vi "PicoScope3000aGetRapidBlock.vi"(0 "error in":errorcluster, 5 "Number of Segments":u32, 7 "handle in":i16, 9 "Device Info":T1, 11 "Rapid Block Acquisition Settings":T2 {"Down Sample Ratio" min=1 step=1; "Down-Sample Mode" items=["None", "Aggregate", "Decimate", "Average"]}) -> (2 "Channel A Buffer":i16[][](array[numeric]), 3 "Channel B Buffer":i16[][](array[numeric]), 4 "error out":errorcluster, 6 "handle out":i16, 8 "noOfSamples Array":u32[](array[numeric]), 10 "Port 0 Buffer":i16[][](array[numeric]), 12 "Overflow":i16[](array[numeric]), 13 "Channel C Buffer":i16[][](array[numeric]), 14 "Channel D Buffer":i16[][](array[numeric]), 15 "Port 1 Buffer":i16[][](array[numeric]))   [LabVIEW 2009]
doc: "This VI gets a set of blocks captured using rapid block mode. It outputs two-dimensional arrays for each channel that contain data from all the requested captures."
uses:
  ps3000a.dll
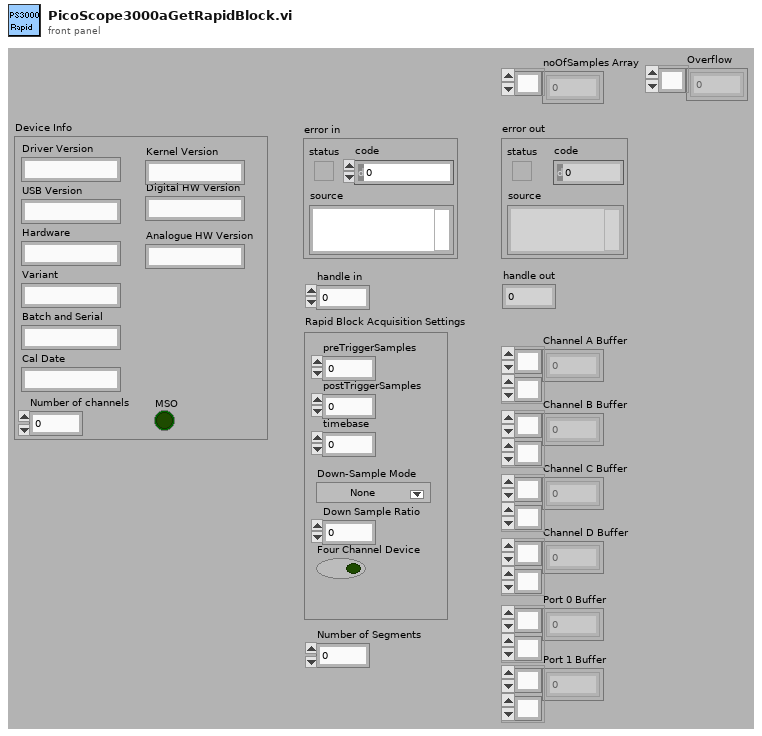
[diagram p1: front panel]
types:
  T1 = cluster{"Driver Version":string, "USB Version":string, "Hardware":string, "Variant":string, "Batch and Serial":string, "Cal Date":string, "Kernel Version":string, "Digital HW Version":string, "Analogue HW Version":string, "MSO":bool, "Number of channels":i16}
  T2 = cluster{"preTriggerSamples":u32, "postTriggerSamples":u32, "timebase":u32, "Down-Sample Mode":i32, "Down Sample Ratio":u32, "Four Channel Device":bool}
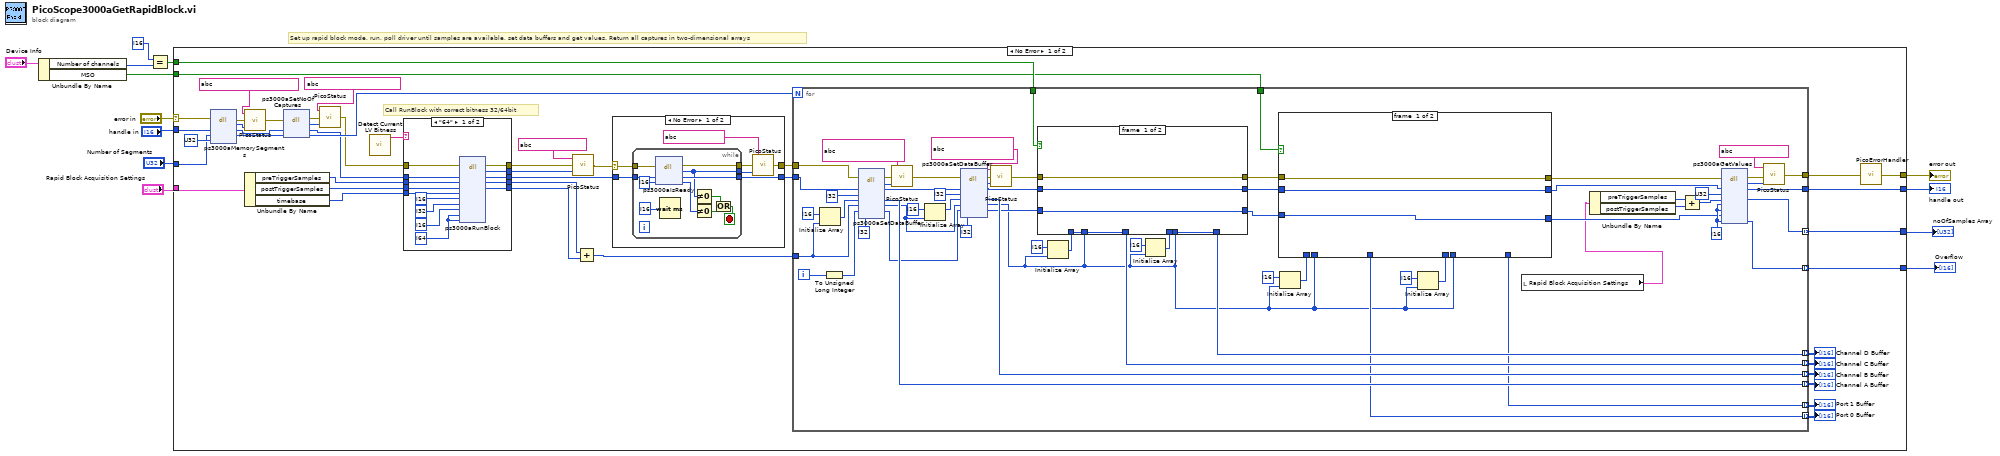
[diagram p0: block diagram]
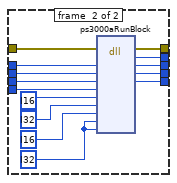
[diagram p2: hidden frame]
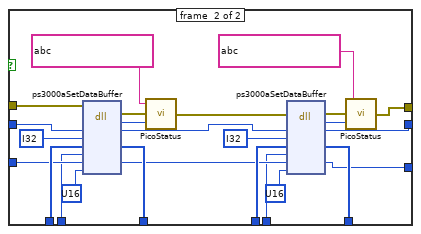
[diagram p3: hidden frame]
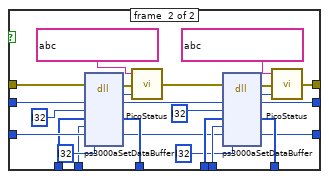
[diagram p4: hidden frame]
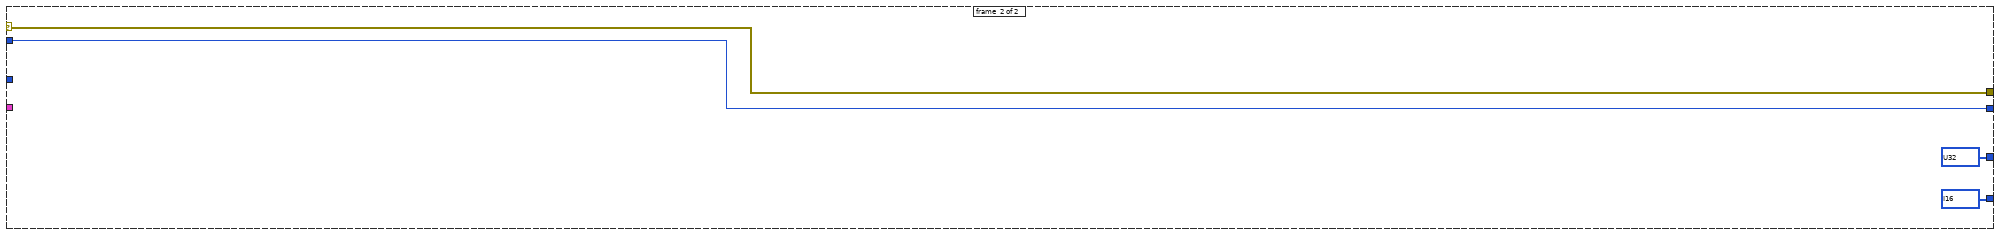
[diagram p6: hidden frame]
diagram:
  # "Set up rapid block mode, run, poll driver until samples are available, set data buffers and get values. Return all captures in two-dimensional arrays"
  n1 = Unbundle By Name("Device Info") -> ("Number of channels"=w8:i16, "MSO"=w5:bool)
  n2 = Equal?(x=i16 ?, y=w8) -> (x = y?=w6:bool)
  n3 = case shown="No Error" "error in" {
    selector: "error in" -> [w53 w229]
    tunnel: [w33 w229] -> w12
    tunnel: "handle in" -> [w52 w228]
    tunnel: [w35 w228] -> w10
    tunnel: [w30 u32[] ?] -> w2
    tunnel: w6 -> [w29 _]
    tunnel: w5 -> [w28 _]
    tunnel: "Rapid Block Acquisition Settings" -> [w27 _]
    tunnel: "Number of Segments" -> [w26 _]
    tunnel: [w14 i16[] ?] -> w1
    frame #0 {
      # "Call RunBlock with correct bitness 32/64bit"
      n4 = dll-call lib="ps3000a.dll" fn="ps3000aMemorySegments" ("ps3000.dll:_ps3000_open_unit@0")(error in=w53, "handle"=w52, "nSegments"=w26, "nMaxSamples"=u32 ?) -> (error out=w50:errorcluster, "PICO_STATUS"=w51:i32, "handle"=w46:i16, "nSegments"=w47:u32)  [unwired: 3 in, 1 out]
      n5 = Unbundle By Name(w27) -> ("preTriggerSamples"=w17:u32, "postTriggerSamples"=w16:u32, "timebase"=w15:u32)
      n6 = call "PicoStatus.vi"("PICO STATUS"=w51, "error in"=w50, "source"=string ?) -> ("error out"=w45:errorcluster)
      n7 = dll-call lib="ps3000a.dll" fn="ps3000aSetNoOfCaptures" ("ps3000.dll:_ps3000_open_unit@0")(error in=w45, "handle"=w46, "nCaptures"=w47) -> (error out=w43:errorcluster, "PICO_STATUS"=w44:i32, "handle"=w18:i16, "nCaptures"=w40:u32)  [unwired: 2 in, 1 out]
      n8 = call "PicoStatus.vi"("PICO STATUS"=w44, "error in"=w43, "source"=string ?) -> ("error out"=w20:errorcluster)
      n9 = call "Detect Current LV Bitness.vi"() -> ("bitness"=w19:string)  [unwired: 11 in]
      n10 = case shown="\"64\"" w19 {
        tunnel: [w71 w85] -> w23
        tunnel: [w70 w84] -> w22
        tunnel: [w69 w83] -> w21
        tunnel: w15 -> [w68 w82]
        tunnel: w17 -> [w67 w81]
        tunnel: w16 -> [w66 w80]
        tunnel: [w65 w79] -> w24
        tunnel: [w64 w78] -> w25
        tunnel: w20 -> [w63 w77]
        tunnel: w18 -> [w62 w76]
        frame #0 {
          w58 = i64 ? ("pParameter")
          n11 = dll-call lib="ps3000a.dll" fn="ps3000aRunBlock" ("ps3000.dll:_ps3000_open_unit@0")(error in=w63, "handle"=w62, "preTriggerSamples"=w67, "postTriggerSamples"=w66, "timebase"=w68, "oversample"=i16 ?, "timeindisposed"=i32 ? ("pParameter"), "segmentIndex"=i16 ? ("pParameter"), "lpReady"=w58, "pParameter"=w58) -> (error out=w64:errorcluster, "PICO_STATUS"=w65:i32, "handle"=w71:i16, "preTriggerSamples"=w70:u32, "postTriggerSamples"=w69:u32)  [unwired: 8 in, 1 out]
        }
        frame #1 {
          w72 = i32 ? ("pParameter")
          n12 = dll-call lib="ps3000a.dll" fn="ps3000aRunBlock" ("ps3000.dll:_ps3000_open_unit@0")(error in=w77, "handle"=w76, "preTriggerSamples"=w81, "postTriggerSamples"=w80, "timebase"=w82, "oversample"=i16 ?, "timeindisposed"=i32 ? ("pParameter"), "segmentIndex"=i16 ? ("pParameter"), "lpReady"=w72, "pParameter"=w72) -> (error out=w78:errorcluster, "PICO_STATUS"=w79:i32, "handle"=w85:i16, "preTriggerSamples"=w84:u32, "postTriggerSamples"=w83:u32)  [unwired: 8 in, 1 out]
        }
      }
      n13 = call "PicoStatus.vi"("PICO STATUS"=w24, "error in"=w25, "source"=string ?) -> ("error out"=w55:errorcluster)
      n14 = Add(x=w22, y=w21) -> (x+y=w41:u32)
      n15 = case shown="No Error" w55 {
        selector: w55 -> [w210 w224]
        tunnel: w23 -> [w212 w225]
        tunnel: [w211 w225] -> w57
        tunnel: [w209 w224] -> w56
        frame #0 {
          n16 = while {
            tunnel: [w223] -> w211
            tunnel: w212 -> [w222]
            tunnel: [w217] -> w207
            tunnel: w210 -> [w216]
            tunnel: [w215] -> w208
            stop <- w221 stop-if-true
            n17 = dll-call lib="ps3000a.dll" fn="ps3000aIsReady" ("ps3000.dll:_ps3000_open_unit@0")(error in=w216, "handle"=w222, "ready"=i16 ?) -> (error out=w215:errorcluster, "status"=w217:i32, "handle"=w223:i16, "ready"=w218:i16)  [unwired: 2 in, 1 out]
            n18 = Wait (ms)(milliseconds to wait=i16 ? ("ready")) -> ()  [unwired: 1 out]
            n19 = Not Equal To 0?(x=w217) -> (x != 0?=w219:bool)
            n20 = Not Equal To 0?(x=w218) -> (x != 0?=w220:bool)
            n21 = Or(x=w219, y=w220) -> (x .or. y?=w221:bool)
          }
          n22 = call "PicoStatus.vi"("PICO STATUS"=w207, "error in"=w208, "source"=string ?) -> ("error out"=w209:errorcluster)
        }
        frame #1 {
        }
      }
      n23 = for {
        N: w40 -> [_]
        tunnel: w57 -> [w147]
        tunnel: w56 -> [w140]
        tunnel: w29 -> [w129]
        tunnel: [w132] -> w39 mode=indexing
        tunnel: [w131] -> w38 mode=indexing
        tunnel: [w110] -> w37 mode=indexing
        tunnel: [w128] -> w36 mode=indexing
        tunnel: w41 -> [w130]
        tunnel: [w119] -> w35
        tunnel: [w105] -> w34
        tunnel: w28 -> [w104]
        tunnel: [w95] -> w32 mode=indexing
        tunnel: [w94] -> w31 mode=indexing
        tunnel: [w88] -> w30 mode=indexing
        tunnel: [w86] -> w14 mode=indexing
        i -> [w90]
        w127 = i16 ? ("overflow")
        n24 = Initialize Array(i16 ? ("element"), w130) -> (w146:i16[])
        n25 = To Unsigned Long Integer(number=w90) -> (unsigned 32bit integer=w89:u32)
        n26 = dll-call lib="ps3000a.dll" fn="ps3000aSetDataBuffer" ("ps3000.dll:_ps3000_open_unit@0")(error in=w140, "handle"=w147, "channel"=i32 ?, "buffer"=w146, "bufferLth"=w130, "waveform"=w89, "downSampleRatioMode"=i32 ?) -> (error out=w138:errorcluster, "PICO_STATUS"=w139:i32, "handle"=w115:i16, "buffer"=w128:i16[], "bufferLth"=w112:i32, "waveform"=w111:u32)  [unwired: 4 in, 1 out]
        n27 = call "PicoStatus.vi"("PICO STATUS"=w139, "error in"=w138, "source"=string ?) -> ("error out"=w116:errorcluster)
        n28 = Initialize Array(i16 ? ("element"), w112) -> (w113:i16[])
        n29 = dll-call lib="ps3000a.dll" fn="ps3000aSetDataBuffer" ("ps3000.dll:_ps3000_open_unit@0")(error in=w116, "handle"=w115, "channel"=i32 ?, "buffer"=w113, "bufferLth"=w112, "waveform"=w111, "downSampleRatioMode"=i32 ?) -> (error out=w118:errorcluster, "PICO_STATUS"=w117:i32, "handle"=w109:i16, "buffer"=w110:i16[], "bufferLth"=w93:i32, "waveform"=w108:u32)  [unwired: 4 in, 1 out]
        n30 = call "PicoStatus.vi"("PICO STATUS"=w117, "error in"=w118, "source"=string ?) -> ("error out"=w137:errorcluster)
        n31 = Initialize Array(i16 ? ("element"), w93) -> (w143:i16[])
        n32 = Initialize Array(i16 ? ("element"), w93) -> (w142:i16[])
        n33 = case shown="True" w129 {
          tunnel: w109 -> [w178 w196]
          tunnel: [w178 w190] -> w100
          tunnel: w143 -> [w180 w198]
          tunnel: w142 -> [w179 w186]
          tunnel: [w179 w192] -> w132
          tunnel: [w180 w200] -> w131
          tunnel: w137 -> [w177 w195]
          tunnel: [w177 w205] -> w103
          tunnel: w93 -> [_ w181]
          tunnel: w93 -> [_ w185]
          tunnel: w108 -> [w176 w199]
          tunnel: [w176 w191] -> w96
          frame #0 {
          }
          frame #1 {
            n34 = dll-call lib="ps3000a.dll" fn="ps3000aSetDataBuffer" ("ps3000.dll:_ps3000_open_unit@0")(error in=w195, "handle"=w196, "channel"=i32 ?, "buffer"=w198, "bufferLth"=w181, "waveform"=w199, "downSampleRatioMode"=i32 ?) -> (error out=w202:errorcluster, "PICO_STATUS"=w201:i32, "handle"=w189:i16, "buffer"=w200:i16[], "waveform"=w184:u32)  [unwired: 5 in, 1 out]
            n35 = call "PicoStatus.vi"("PICO STATUS"=w201, "error in"=w202, "source"=string ?) -> ("error out"=w188:errorcluster)
            n36 = dll-call lib="ps3000a.dll" fn="ps3000aSetDataBuffer" ("ps3000.dll:_ps3000_open_unit@0")(error in=w188, "handle"=w189, "channel"=i32 ?, "buffer"=w186, "bufferLth"=w185, "waveform"=w184, "downSampleRatioMode"=i32 ?) -> (error out=w194:errorcluster, "PICO_STATUS"=w193:i32, "handle"=w190:i16, "buffer"=w192:i16[], "waveform"=w191:u32)  [unwired: 5 in, 1 out]
            n37 = call "PicoStatus.vi"("PICO STATUS"=w193, "error in"=w194, "source"=string ?) -> ("error out"=w205:errorcluster)
          }
        }
        n38 = Initialize Array(i16 ? ("element"), w93) -> (w97:i16[])
        n39 = Initialize Array(i16 ? ("element"), w93) -> (w92:i16[])
        n40 = case shown="True" w104 {
          tunnel: w103 -> [w150 w175]
          tunnel: w100 -> [w149 w174]
          tunnel: w97 -> [_ w172]
          tunnel: w93 -> [_ w152]
          tunnel: w92 -> [_ w170]
          tunnel: [_ w169] -> w95
          tunnel: [_ w168] -> w94
          tunnel: [w149 w162] -> w101
          tunnel: [w150 w161] -> w102
          tunnel: w96 -> [w148 w156]
          tunnel: w93 -> [_ w154]
          tunnel: [w148 w151] -> w91
          frame #0 {
          }
          frame #1 {
            n41 = dll-call lib="ps3000a.dll" fn="ps3000aSetDataBuffer" ("ps3000.dll:_ps3000_open_unit@0")(error in=w175, "handle"=w174, "channel"=i32 ?, "buffer"=w172, "bufferLth"=w154, "segmentIndex"=w156, "mode"=u16 ? ("segmentIndex")) -> (error out=w166:errorcluster, "PICO_STATUS"=w167:i32, "handle"=w160:i16, "buffer"=w169:i16[], "segmentIndex"=w155:u32)  [unwired: 5 in, 1 out]
            n42 = call "PicoStatus.vi"("PICO STATUS"=w167, "error in"=w166, "source"=string ?) -> ("error out"=w163:errorcluster)
            n43 = dll-call lib="ps3000a.dll" fn="ps3000aSetDataBuffer" ("ps3000.dll:_ps3000_open_unit@0")(error in=w163, "handle"=w160, "channel"=i32 ?, "buffer"=w170, "bufferLth"=w152, "segmentIndex"=w155, "mode"=u16 ? ("segmentIndex")) -> (error out=w164:errorcluster, "PICO_STATUS"=w165:i32, "handle"=w162:i16, "buffer"=w168:i16[], "segmentIndex"=w151:u32)  [unwired: 5 in, 1 out]
            n44 = call "PicoStatus.vi"("PICO STATUS"=w165, "error in"=w164, "source"=string ?) -> ("error out"=w161:errorcluster)
          }
        }
        n45 = local read "Rapid Block Acquisition Settings"() -> (w87:T2)
        n46 = Unbundle By Name(w87) -> ("preTriggerSamples"=w125:u32, "postTriggerSamples"=w124:u32)
        n47 = Add(x=w125, y=w124) -> (x+y=w126:u32)
        n48 = dll-call lib="ps3000a.dll" fn="ps3000aGetValues" ("ps3000.dll:_ps3000_open_unit@0")(error in=w102, "handle"=w101, "startIndex"=u32 ?, "noOfSamples"=w126, "downSampleRatio"=w127, "downSampleRatioMode"=w127, "segmentIndex"=w91, "overflow"=w127) -> (error out=w121:errorcluster, "PICO_STATUS"=w120:i32, "handle"=w119:i16, "noOfSamples"=w88:u32, "overflow"=w86:i16)  [unwired: 6 in, 1 out]
        n49 = call "PicoStatus.vi"("PICO STATUS"=w120, "error in"=w121, "source"=string ?) -> ("error out"=w105:errorcluster)
      }
      "Channel D Buffer" <- w39
      "Channel C Buffer" <- w38
      "Channel B Buffer" <- w37
      "Channel A Buffer" <- w36
      "Port 0 Buffer" <- w32
      "Port 1 Buffer" <- w31
      n50 = call "PicoErrorHandler.vi"("error in"=w34) -> ("error out"=w33:errorcluster)
    }
    frame #1 {
    }
  }
  "error out" <- w12
  "handle out" <- w10
  "noOfSamples Array" <- w2
  "Overflow" <- w1
